vi "y_axis_stepper_motor.vi"(8 "speed":u32(knob) scale=0.0..20.0, 11 "Direction":bool[](array[boolean])) -> ()   [LabVIEW 2016]
uses:
  <vilib>/DigilentWF/DigilentWF.lvlib
panel:
  # "This program is turn y-axis stepper motor with one step only.\n The y-axis is axis is from or towards the egg's poles.\nThis stepper motor driven by a A4988 driver with 1/16 resolution.  \nThe  digital I/O pin 8 of Analog Discovery 2 is connected to the enable pin of A4988 driver with implement low logic level.\nThe  digital I/O pin 9 of Analog Discovery 2 is connected to the step pin of A4988 driver with implement a pulse.\nThe  digital I/O pin 10 of Analog Discovery 2 is connected to the direction pin of A4988 driver the value will be input the by user (low logic level or high logic lovel).\nThe  digital I/O pin 11 to 13 of Analog Discovery 2 is connected to the mirco-stepping pin of A4988 driver with implement the all high logic lovel."
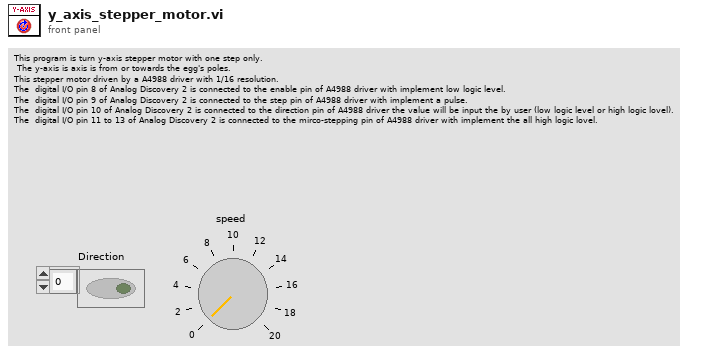
[diagram p1: front panel]
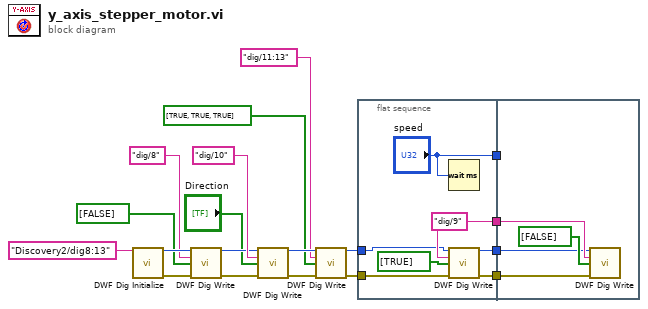
[diagram p0: block diagram]
diagram:
  n1 = call <vilib>:"DWF Dig Initialize.vi"("Device Name/Lines"="Discovery2/dig8:13") -> ("Instrument Handle Out"=w14:u32, "Error Out"=w13:errorcluster)  [unwired: 13 in]
  n2 = call <vilib>:"DWF Dig Write.vi"("Instrument Handle In"=w14, "Lines"="dig/8" ("Disable line"), "Data"=bool[] [FALSE] ("disable"), "Error In"=w13) -> ("Instrument Handle Out"=w10:u32, "Error Out"=w9:errorcluster)  [unwired: 10 in]
  n3 = call <vilib>:"DWF Dig Write.vi"("Instrument Handle In"=w10, "Lines"="dig/10" ("Direction line"), "Data"="Direction", "Error In"=w9) -> ("Instrument Handle Out"=w8:u32, "Error Out"=w7:errorcluster)  [unwired: 10 in]
  n4 = call <vilib>:"DWF Dig Write.vi"("Instrument Handle In"=w8, "Lines"="dig/11:13" ("Microstepping line"), "Data"=bool[] [TRUE, TRUE, TRUE] ("microstepping"), "Error In"=w7) -> ("Instrument Handle Out"=w6:u32, "Error Out"=w5:errorcluster)  [unwired: 10 in]
  n5 = flat-sequence {
    tunnel: [w25] -> w19
    tunnel: w6 -> [w24]
    tunnel: w5 -> [w23]
    tunnel: [w22] -> w18
    tunnel: [w21] -> w17
    tunnel: ["speed"] -> w16
    tunnel: w19 -> [w29]
    tunnel: w18 -> [w28]
    tunnel: w17 -> [w27]
    tunnel: w16 -> [_]
    frame #0 {
      w25 = "dig/9" ("Step line")
      n6 = Wait (ms)(milliseconds to wait="speed") -> ()  [unwired: 1 out]
      n7 = call <vilib>:"DWF Dig Write.vi"("Instrument Handle In"=w24, "Lines"=w25, "Data"=bool[] [TRUE], "Error In"=w23) -> ("Instrument Handle Out"=w21:u32, "Error Out"=w22:errorcluster)  [unwired: 10 in]
    }
    frame #1 {
      n8 = call <vilib>:"DWF Dig Write.vi"("Instrument Handle In"=w27, "Lines"=w29, "Data"=bool[] [FALSE], "Error In"=w28) -> ()  [unwired: 10 in, 2 out]
    }
  }
